vi "Online_OneClick.vi"() -> ()   [LabVIEW 2014]
uses:
  <vilib>/Utility/file.llb/Read From Spreadsheet File (string).vi
panel:
  in  "Online_Values":path
  in  "개별 Training":path
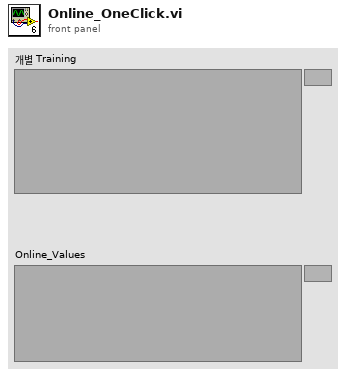
[diagram p1: front panel]
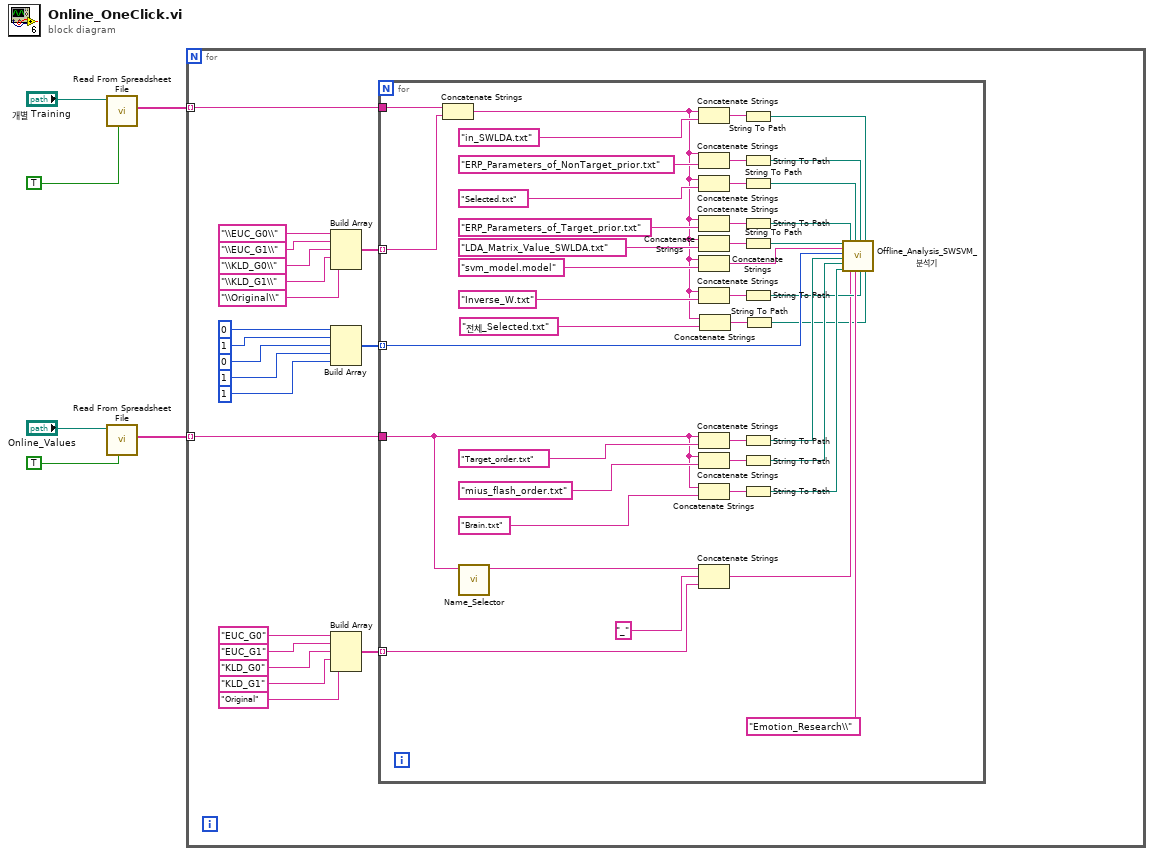
[diagram p0: block diagram]
diagram:
  n1 = call-poly <vilib>:"Read From Spreadsheet File.vi"("transpose (no:F)"=TRUE, "file path (dialog if empty)"="개별 Training") -> ("first row"=w4:string[])  [unwired: 5 in, 4 out]
  n2 = call-poly <vilib>:"Read From Spreadsheet File.vi"("transpose (no:F)"=TRUE, "file path (dialog if empty)"="Online_Values") -> ("first row"=w1:string[])  [unwired: 5 in, 4 out]
  n3 = for {
    tunnel: w4 -> [w20] mode=indexing
    tunnel: w1 -> [w19] mode=indexing
    n4 = Build Array("\\EUC_G0\\", "\\EUC_G1\\", "\\KLD_G0\\", "\\KLD_G1\\", "\\Original\\") -> (w22:string[])
    n5 = Build Array(0, 1, 0, 1, 1) -> (w13:i32[])
    n6 = Build Array("EUC_G0", "EUC_G1", "KLD_G0", "KLD_G1", "Original") -> (w7:string[])
    n7 = for {
      tunnel: w22 -> [w66] mode=indexing
      tunnel: w20 -> [w67]
      tunnel: w19 -> [w43]
      tunnel: w13 -> [w42] mode=indexing
      tunnel: w7 -> [w32] mode=indexing
      n8 = Concatenate Strings(w67, w66) -> (w28:string)
      n9 = call "Name_Selector.vi"("Path"=w43) -> ("Name"=w33:string)  [unwired: 10 in]
      n10 = Concatenate Strings(w28, "in_SWLDA.txt") -> (w59:string)
      n11 = Concatenate Strings(w28, "ERP_Parameters_of_NonTarget_prior.txt") -> (w63:string)
      n12 = Concatenate Strings(w28, "Selected.txt") -> (w41:string)
      n13 = Concatenate Strings(w28, "ERP_Parameters_of_Target_prior.txt") -> (w54:string)
      n14 = Concatenate Strings(w28, "LDA_Matrix_Value_SWLDA.txt") -> (w56:string)
      n15 = Concatenate Strings(w28, "svm_model.model") -> (w37:string)
      n16 = Concatenate Strings(w28, "Inverse_W.txt") -> (w36:string)
      n17 = Concatenate Strings(w43, "Target_order.txt") -> (w52:string)
      n18 = Concatenate Strings(w43, "mius_flash_order.txt") -> (w49:string)
      n19 = Concatenate Strings(w43, "Brain.txt") -> (w47:string)
      n20 = Concatenate Strings(w33, "_" ("string"), w32) -> (w34:string)
      n21 = Concatenate Strings(w28, "전체_Selected.txt") -> (w30:string)
      n22 = String To Path(string=w59) -> (path=w58:path)
      n23 = String To Path(string=w63) -> (path=w62:path)
      n24 = String To Path(string=w41) -> (path=w40:path)
      n25 = String To Path(string=w54) -> (path=w61:path)
      n26 = String To Path(string=w56) -> (path=w55:path)
      n27 = String To Path(string=w36) -> (path=w35:path)
      n28 = String To Path(string=w52) -> (path=w51:path)
      n29 = String To Path(string=w49) -> (path=w48:path)
      n30 = String To Path(string=w47) -> (path=w46:path)
      n31 = String To Path(string=w30) -> (path=w27:path)
      n32 = call "Offline_Analysis_SWSVM_분석기.vi"("LDA_matrix"=w55, "svm_model_file"=w37, "Group Number"=w42, "Target_order.txt"=w51, "mius_flash_order"=w48, "Brain"=w46, "Target"=w61, "피험자이름"=w34, "Selected"=w40, "Save_path"="Emotion_Research\\", "Nontarget"=w62, "W"=w35, "in_matrix"=w58, "전체_Selected"=w27) -> ()  [unwired: 6 in]
    }
  }
